vi "Set Required Objects.vi"(8 "error in":errorcluster, 10 "Required Objects":set{T1}(c389), 11 "Device Profile in":refnum<class "Device Profile.lvclass">) -> (0 "error out":errorcluster, 3 "Device Profile out":refnum<class "Device Profile.lvclass">)   [LabVIEW 2020, in "CANopen.lvlib" / "Device Profile.lvclass"]
uses:
  Device Profile.lvclass
  Device Profile.lvclass/Device Profile.ctl
  Typedefs/Data Type.ctl
  CANopen.lvlib
  Typedefs/OD Entry Spec.ctl
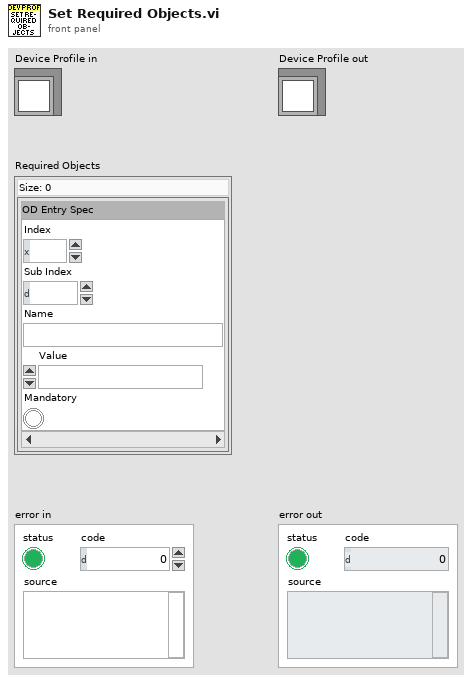
[diagram p1: front panel]
types:
  T1 = typedef "CANopen.lvlib/OD Entry Spec.ctl" = cluster{"Index":u16, "Sub Index":u8, "Name":string, "Value":T2, "Mandatory":bool}
  T2 = typedef "CANopen.lvlib/Data Type.ctl" = u16
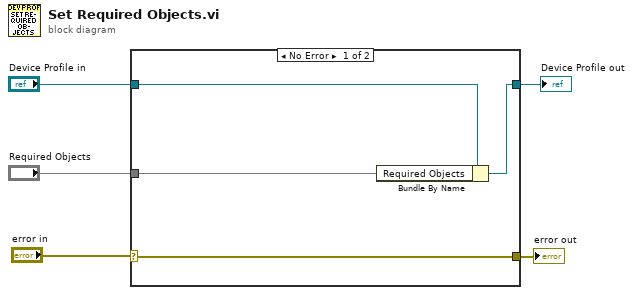
[diagram p0: block diagram]
diagram:
  n1 = case shown="No Error" "error in" {
    selector: "error in" -> [w9 w10]
    tunnel: [w9 w10] -> w2
    tunnel: [w7 w11] -> w4
    tunnel: "Device Profile in" -> [w8 w11]
    tunnel: "Required Objects" -> [w6 _]
    frame No Error {
      n2 = Bundle By Name(cluster=w8, "Required Objects"=w6) -> (w7:refnum<class "Device Profile.lvclass">)
    }
    frame Error {
    }
  }
  "error out" <- w2
  "Device Profile out" <- w4
